vi "controller.vi"() -> ()   [LabVIEW 2020]
uses:
  <vilib>/Utility/file.llb/Write Delimited Spreadsheet (string).vi
panel:
  in  "stop":bool
  in  "error in (no error)":errorcluster
  in  "VISA resource name":refnum<visa-resource-name>
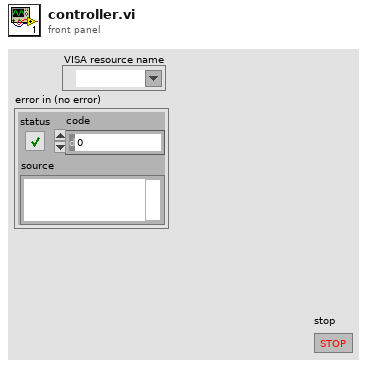
[diagram p1: front panel]
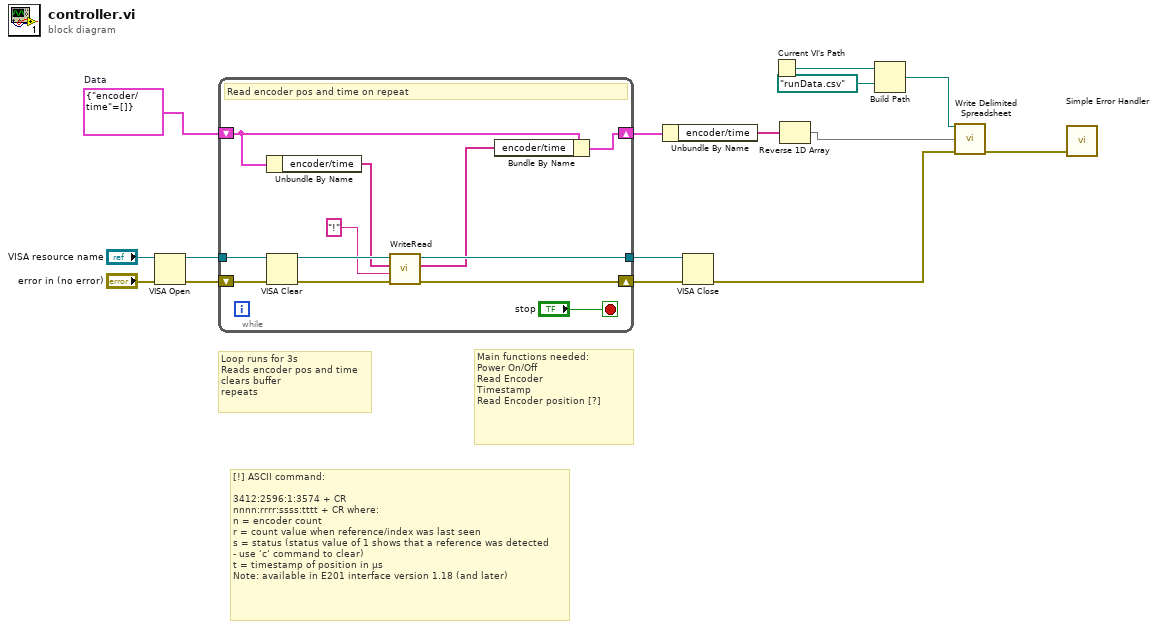
[diagram p0: block diagram]
diagram:
  w11 = cluster{"encoder/time":string[]} {"encoder/time"=[]}  # Data
  # "[!] ASCII command:\n\n3412:2596:1:3574 + CR\nnnnn:rrrr:ssss:tttt + CR where:\nn = encoder count\nr = count value when reference/index was last seen\ns = status (status value of 1 shows that a reference was detected\n- use ‘c’ command to clear)\nt = timestamp of position in µs\nNote: available in E201 interface version 1.18 (and later)"
  # "Loop runs for 3s\nReads encoder pos and time\nclears buffer\nrepeats"
  # "Main functions needed:\nPower On/Off\nRead Encoder\nTimestamp \nRead Encoder position [?]"
  n1 = VISA Open(error in (no error)="error in (no error)", VISA resource name="VISA resource name") -> (VISA resource name=w12:refnum<visa-resource-name>, error out=w13:errorcluster)  [unwired: 3 in]
  n2 = while {
    tunnel: w12 -> [w26]
    shift-right: [w21] -> w9
    shift-left: w11 -> [w22]
    shift-right: [w18] -> w10
    shift-left: w13 -> [w27]
    tunnel: [w19] -> w8
    stop <- "stop" stop-if-true
    # "Read encoder pos and time on repeat"
    n3 = Unbundle By Name "Unbundle By Name"(w22) -> ("encoder/time"=w16:string[])
    n4 = VISA Clear(VISA resource name=w26, error in (no error)=w27) -> (VISA resource name out=w24:refnum<visa-resource-name>, error out=w25:errorcluster)
    n5 = call "WriteRead.vi"("error in (no error)"=w25, "write buffer"="!", "Data in"=w16, "VISA Refnum in"=w24) -> ("error out"=w18:errorcluster, "Data out"=w17:string[], "VISA resource name out"=w19:refnum<visa-resource-name>)  [unwired: 5 in]
    n6 = Bundle By Name(cluster=w22, "encoder/time"=w17) -> (w21:cluster{"encoder/time":string[]})
  }
  n7 = Unbundle By Name(w9) -> ("encoder/time"=w2:string[])
  n8 = VISA Close(VISA resource name=w8, error in (no error)=w10) -> (error out=w7:errorcluster)
  n9 = Current VI's Path() -> (path=w6:path)
  n10 = Reverse 1D Array(array=w2) -> (reversed array=w1:string[])
  n11 = Build Path(base path=w6, name or relative path=path "runData.csv") -> (appended path=w4:path)
  n12 = call-poly <vilib>:"Write Delimited Spreadsheet.vi"("file path (dialog if empty)"=w4, "1D data"=w1, "error in (no error)"=w7) -> ("error out"=w3:errorcluster)  [unwired: 11 in, 1 out]
  n13 = call <vilib>:"Simple Error Handler.vi"("error in (no error)"=w3) -> ()  [unwired: 4 in, 5 out]
